vi "8BitFullAdder.vi"() -> ()   [LabVIEW 2015]
panel:
  out "Output":u8
  out "OutputArray":bool[](array[boolean])
  out "Inp2BooleanArray":bool[](array[boolean])
  out "Inp1BooleanArray":bool[](array[boolean])
  in  "Inp2":u8
  in  "Inp1":u8
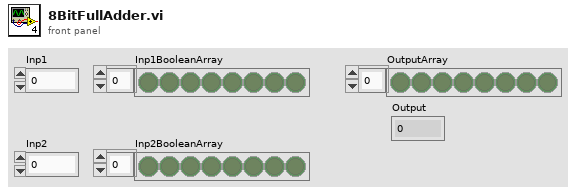
[diagram p1: front panel]
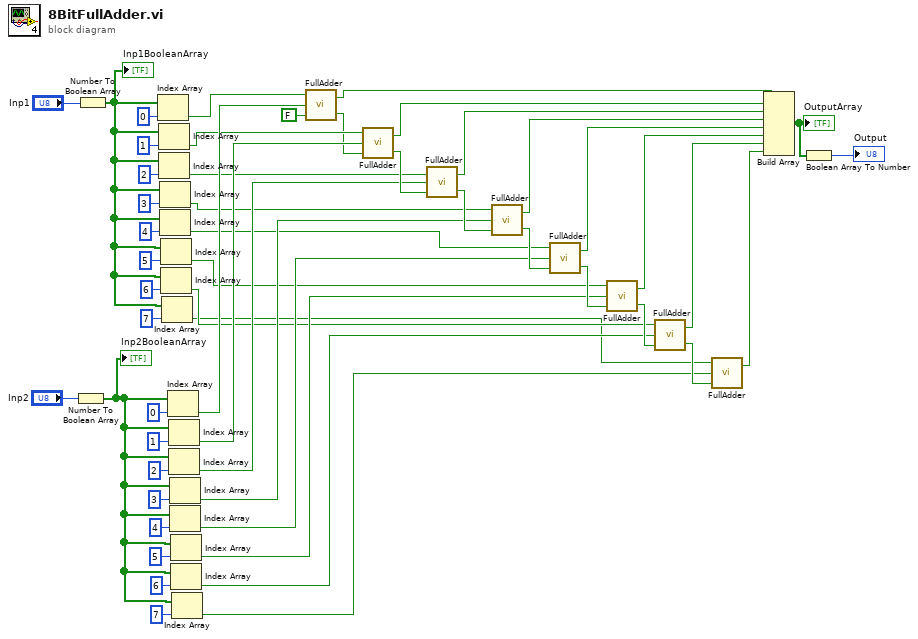
[diagram p0: block diagram]
diagram:
  n1 = Number To Boolean Array(number="Inp2") -> (Boolean array=w35:bool[])
  "Inp2BooleanArray" <- w35
  n2 = Number To Boolean Array(number="Inp1") -> (Boolean array=w44:bool[])
  "Inp1BooleanArray" <- w44
  n3 = Index Array(array=w44, index=0) -> (element=w34:bool)
  n4 = Index Array(array=w44, index=1) -> (element=w31:bool)
  n5 = Index Array(array=w44, index=2) -> (element=w22:bool)
  n6 = Index Array(array=w44, index=3) -> (element=w20:bool)
  n7 = Index Array(array=w44, index=4) -> (element=w18:bool)
  n8 = Index Array(array=w44, index=5) -> (element=w16:bool)
  n9 = Index Array(array=w44, index=6) -> (element=w14:bool)
  n10 = Index Array(array=w44, index=7) -> (element=w12:bool)
  n11 = Index Array(array=w35, index=0) -> (element=w33:bool)
  n12 = Index Array(array=w35, index=1) -> (element=w30:bool)
  n13 = Index Array(array=w35, index=2) -> (element=w21:bool)
  n14 = Index Array(array=w35, index=3) -> (element=w19:bool)
  n15 = Index Array(array=w35, index=4) -> (element=w17:bool)
  n16 = Index Array(array=w35, index=5) -> (element=w15:bool)
  n17 = Index Array(array=w35, index=6) -> (element=w13:bool)
  n18 = Index Array(array=w35, index=7) -> (element=w11:bool)
  n19 = call "FullAdder.vi"("Cin"=FALSE, "B"=w33, "A"=w34) -> ("Cout"=w29:bool, "S"=w10:bool)
  n20 = call "FullAdder.vi"("Cin"=w29, "B"=w30, "A"=w31) -> ("Cout"=w28:bool, "S"=w9:bool)
  n21 = call "FullAdder.vi"("Cin"=w28, "B"=w21, "A"=w22) -> ("Cout"=w27:bool, "S"=w8:bool)
  n22 = call "FullAdder.vi"("Cin"=w27, "B"=w19, "A"=w20) -> ("Cout"=w26:bool, "S"=w7:bool)
  n23 = call "FullAdder.vi"("Cin"=w26, "B"=w17, "A"=w18) -> ("Cout"=w25:bool, "S"=w6:bool)
  n24 = call "FullAdder.vi"("Cin"=w25, "B"=w15, "A"=w16) -> ("Cout"=w24:bool, "S"=w5:bool)
  n25 = call "FullAdder.vi"("Cin"=w24, "B"=w13, "A"=w14) -> ("Cout"=w23:bool, "S"=w4:bool)
  n26 = call "FullAdder.vi"("Cin"=w23, "B"=w11, "A"=w12) -> ("S"=w3:bool)  [unwired: 1 out]
  n27 = Build Array(w10, w9, w8, w7, w6, w5, w4, w3) -> (w2:bool[])
  "OutputArray" <- w2
  n28 = Boolean Array To Number(Boolean array=w2) -> (number=→"Output":u32)
